vi "UTF-8 To Encoded String.vi"(8 "error in (no error)":errorcluster, 10 "UTF-8 string":string, 11 "Encoding in":refnum<class "CConfig UCS-16 Encoding.lvclass">) -> (0 "error out":errorcluster, 2 "Encoded string":string, 3 "Encoding out":refnum<class "CConfig UCS-16 Encoding.lvclass">)   [LabVIEW 2013, in "CConfig UCS-16 Encoding.lvclass"]
doc: "Copyright 2018, Carya Automatisering, Wiebe Walstra."
uses:
  CConfig UCS-16 Encoding.lvclass
  CConfig UCS-16 Encoding.lvclass/CConfig UCS-16 Encoding.ctl
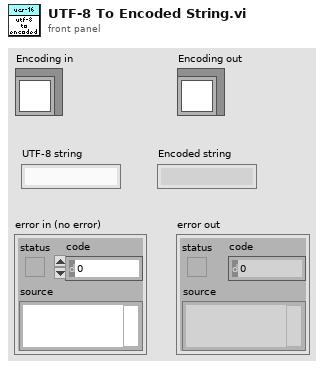
[diagram p1: front panel]
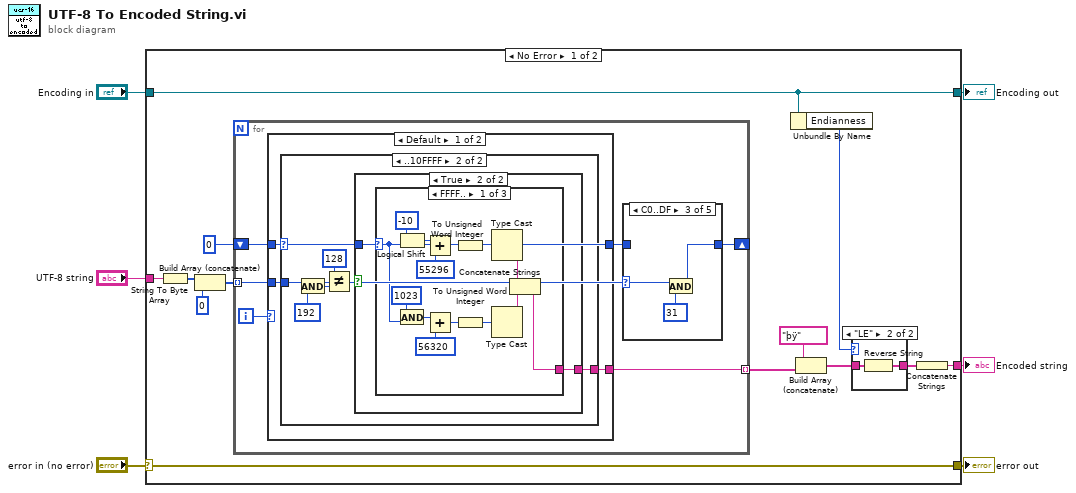
[diagram p0: block diagram]
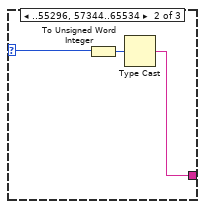
[diagram p5: hidden frame]
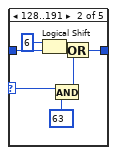
[diagram p9: hidden frame]
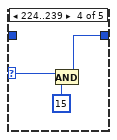
[diagram p10: hidden frame]
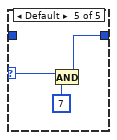
[diagram p11: hidden frame]
diagram:
  n1 = case shown="No Error" "error in (no error)" {
    selector: "error in (no error)" -> [w11 w77]
    tunnel: [w13 w78] -> w2
    tunnel: "UTF-8 string" -> [w12 w78]
    tunnel: [w11 w77] -> w1
    tunnel: "Encoding in" -> [w10 w76]
    tunnel: [w10 w76] -> w3
    frame No Error {
      n2 = String To Byte Array(string=w12) -> (unsigned byte array=w19:u8[])
      n3 = Build Array (concatenate)(w19, u8 0) -> (w16:u8[])
      n4 = for {
        tunnel: w16 -> [w24] mode=indexing
        shift-right: [w28] -> _
        shift-left: u32 0 -> [w25]
        tunnel: [w23] -> w17 mode=indexing
        i -> [w27]
        n5 = case shown="Default" w27 {
          tunnel: [w30 w58] -> w26
          tunnel: w25 -> [w30 w58]
          tunnel: w24 -> [w31 _]
          tunnel: [w29 _] -> w23
          frame Default {
            n6 = case shown="..10FFFF" w30 {
              selector: w30 -> [_ w33]
              tunnel: w31 -> [_ w37]
              tunnel: [_ w32] -> w29
              frame Default {
              }
              frame ..1114111 {
                n7 = And(x=w37, y=u8 192) -> (x .and. y?=w36:u8)
                n8 = Not Equal?(x=u8 128 ("y"), y=w36) -> (x != y?=w34:bool)
                n9 = case shown="True" w34 {
                  tunnel: w33 -> [_ w40]
                  tunnel: [_ w39] -> w32
                  frame False {
                  }
                  frame True {
                    n10 = case shown="FFFF.." w40 {
                      selector: w40 -> [w45 w56 _]
                      tunnel: [w41 w55 _] -> w39
                      frame 65535.. {
                        n11 = Logical Shift(y=i16 -10, x=w45) -> (x << y=w53:u32)
                        n12 = And(x=u16 1023 ("y"), y=w45) -> (x .and. y?=w46:u32)
                        n13 = Add(x=w53, y=u16 55296) -> (x+y=w51:u32)
                        n14 = Add(x=w46, y=u16 56320) -> (x+y=w48:u32)
                        n15 = To Unsigned Word Integer(number=w51) -> (unsigned 16bit integer=w50:u16)
                        n16 = To Unsigned Word Integer(number=w48) -> (unsigned 16bit integer=w49:u16)
                        n17 = Type Cast(x=w50) -> (*(type *) &x=w43:string)  [unwired: 1 in]
                        n18 = Type Cast(x=w49) -> (*(type *) &x=w42:string)  [unwired: 1 in]
                        n19 = Concatenate Strings(w43, w42) -> (w41:string)
                      }
                      frame ..55296, 57344..65534 {
                        n20 = To Unsigned Word Integer(number=w56) -> (unsigned 16bit integer=w57:u16)
                        n21 = Type Cast(x=w57) -> (*(type *) &x=w55:string)  [unwired: 1 in]
                      }
                      frame Default {
                      }
                    }
                  }
                }
              }
            }
          }
          frame 0 {
          }
        }
        n22 = case shown="C0..DF" w24 {
          selector: w24 -> [w59 w62 w69 w72 w75]
          tunnel: w26 -> [_ w64 _ _ _]
          tunnel: [w59 w63 w67 w70 w73] -> w28
          frame ..127 {
          }
          frame 128..191 {
            n23 = Logical Shift(y=i16 6, x=w64) -> (x << y=w66:u32)
            n24 = And(x=w62, y=u8 63) -> (x .and. y?=w60:u8)
            n25 = Or(x=w66, y=w60) -> (x .or. y?=w63:u32)
          }
          frame 192..223 {
            n26 = And(x=w69, y=u8 31) -> (x .and. y?=w67:u8)
          }
          frame 224..239 {
            n27 = And(x=w72, y=u8 15) -> (x .and. y?=w70:u8)
          }
          frame Default {
            n28 = And(x=w75, y=u8 7) -> (x .and. y?=w73:u8)
          }
        }
      }
      n29 = Unbundle By Name(w10) -> ("Endianness"=w9:enum16{"BE", "LE", "unknown"})
      n30 = Build Array (concatenate)("þÿ" ("true string"), w17) -> (w8:string[])
      n31 = case shown="\"LE\"" w9 {
        tunnel: w8 -> [w20 w22]
        tunnel: [w20 w21] -> w14
        frame "BE", Default {
        }
        frame "LE" {
          n32 = Reverse String(1:w22) -> (0:w21:string[])
        }
      }
      n33 = Concatenate Strings(w14) -> (w13:string)
    }
    frame Error {
    }
  }
  "error out" <- w1
  "Encoding out" <- w3
  "Encoded string" <- w2
